vi "SFC_Change Pallet.vi"(5 "TYN":string, 6 "strUserID":string, 7 "strNewPalletID":string, 8 "error in (no error)":errorcluster caption="错误输入（无错误）", 9 "stroldBOXID":string, 10 "strSID":string, 11 "Traceability 引用句柄":refnum<k24>) -> (0 "error out":errorcluster caption="错误输出", 2 "SFC_ChangePallet":string, 3 "Traceability 引用句柄输出":refnum<k24>)   [LabVIEW 2014, in "Traceability.lvlib"]
uses:
  D:/webservice/Traceability.dll
  Traceability.dll
  Traceability.lvlib
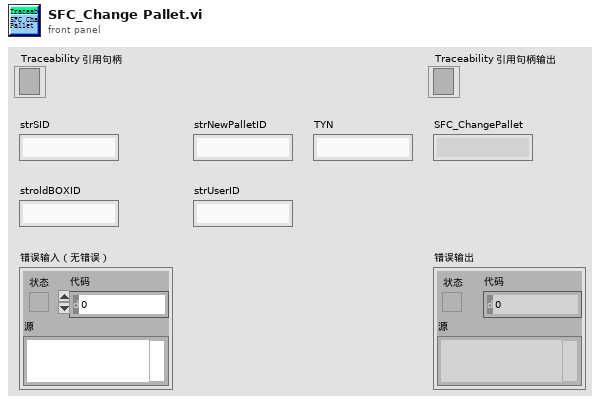
[diagram p1: front panel]
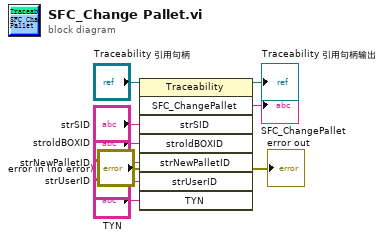
[diagram p0: block diagram]
diagram:
  n1 = invoke class="Traceability" method="SFC_ChangePallet"(reference="Traceability 引用句柄", error in="error in (no error)", "strSID"="strSID", "stroldBOXID"="stroldBOXID", "strNewPalletID"="strNewPalletID", "strUserID"="strUserID", "TYN"="TYN") -> (reference out=→"Traceability 引用句柄输出":refnum<k24>, error out=→"error out":errorcluster, "SFC_ChangePallet"=→"SFC_ChangePallet":string)  [unwired: 1 in, 5 out]
